vi "GPIBReadTemp.vi"(1 "GPIB Address":string="9") -> (0 "Temp":dbl format="%.2f")   [LabVIEW 2016]
doc: "A device connected to a GPIB bus can be written to or be read from using this VI. Select the GPIB address of the device, choose Read or Write or both, type in the characters to be written, and run the VI. If you choose both Read and Write, the VI will write to the device first, then read from the device. Before using this VI you should initialize the GPIB address according to the device's specifications with the \"GPIB Initialization\" function."
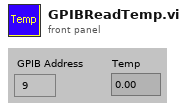
[diagram p1: front panel]
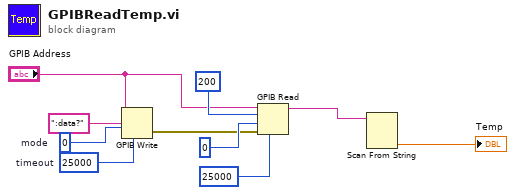
[diagram p0: block diagram]
diagram:
  w8 = u32 25000  # timeout
  w10 = 0  # mode
  n1 = GPIB Write(0:"GPIB Address", 1:":data?" ("Characters to Write"), 2:w10, 4:w8) -> (6:w3:errorcluster)  [unwired: 1 in, 1 out]
  n2 = GPIB Read(0:"GPIB Address", 1:200 ("# bytes\nto read"), 2:0 ("mode"), 3:w3, 4:u32 25000 ("timeout")) -> (5:w2:string)  [unwired: 2 out]
  n3 = Scan From String(input string=w2) -> (output 1=→"Temp":dbl)  [unwired: 4 in, 3 out]
